vi "Metadata check for empty fields.vi"(8 "error in (no error)":errorcluster, 10 "Output Path":path, 11 "Control references":refnum<vi>[](array[refnum])) -> (0 "error out":errorcluster, 2 "Missing Field":bool, 3 "Field Names":string[](array[string]))   [LabVIEW 2014, in "Metadata.lvlib"]
uses:
  Metadata.lvlib
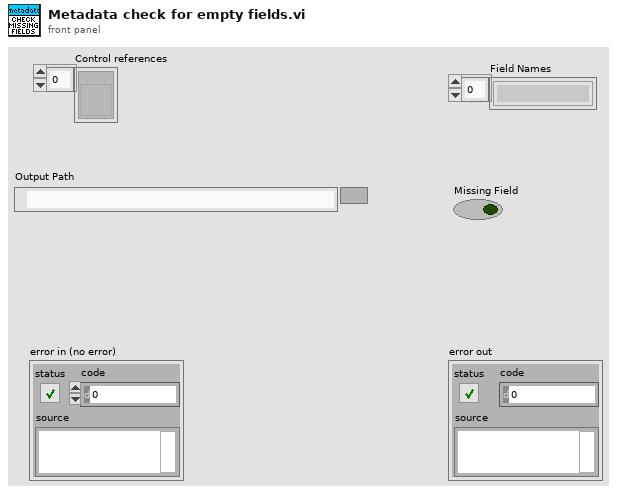
[diagram p1: front panel]
types:
  T1 = enum8{"Enabled", "Disabled", "Disabled and Grayed Out"}
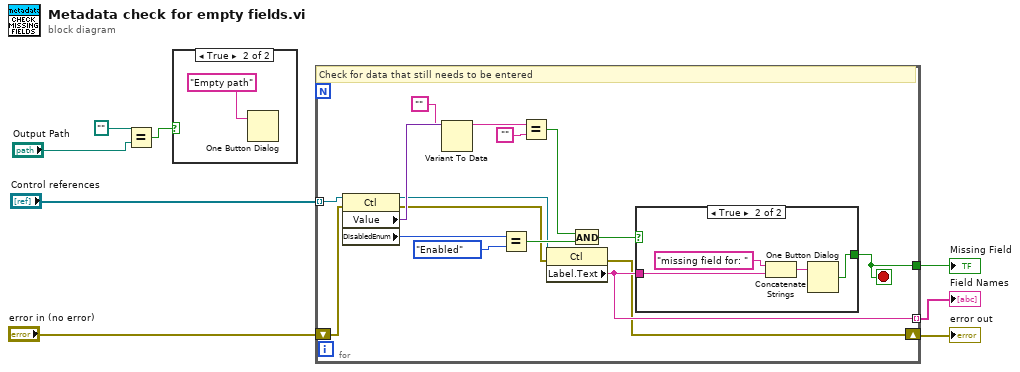
[diagram p0: block diagram]
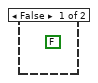
[diagram p2: hidden frame]
diagram:
  n1 = Equal?(x=path "", y="Output Path") -> (x = y?=w2:bool)
  n2 = case shown="True" w2 {
    frame False {
      (unwired) FALSE ("true")
    }
    frame True {
      n3 = One Button Dialog(message="Empty path") -> ()  [unwired: 1 in, 1 out]
    }
  }
  n4 = for {
    tunnel: [w25] -> w5
    tunnel: [w20] -> w4 mode=indexing
    shift-right: [w13] -> w7
    shift-left: "error in (no error)" -> [w12]
    tunnel: "Control references" -> [w11] mode=indexing
    stop <- w25 stop-if-true
    # "Check for data that still needs to be entered"
    n5 = property class="Ctl"(reference=w11, error in=w12) -> (reference out=w10:refnum<vi>, error out=w14:errorcluster, "Value"=w24:variant, "DisabledEnum"=w19:T1)
    n6 = Variant To Data(type="", Variant=w24) -> (data=w23:string)  [unwired: 1 in, 1 out]
    n7 = Equal?(x=w19, y=T1."Enabled" ("Disabled")) -> (x = y?=w15:bool)
    n8 = Equal?(x=w23, y="") -> (x = y?=w17:bool)
    n9 = property class="Ctl"(reference=w10, error in=w14) -> (error out=w13:errorcluster, "Label.Text"=w20:string)  [unwired: 1 out]
    n10 = And(x=w17, y=w15) -> (x .and. y?=w16:bool)
    n11 = case shown="True" w16 {
      selector: w16 -> [w26 _]
      tunnel: w20 -> [_ w29]
      tunnel: [w26 w27] -> w25
      frame False {
      }
      frame True {
        n12 = Concatenate Strings("missing field for: ", w29) -> (w28:string)
        n13 = One Button Dialog(message=w28) -> (true=w27:bool)  [unwired: 1 in]
      }
    }
  }
  "error out" <- w7
  "Missing Field" <- w5
  "Field Names" <- w4
